vi "Best_EXP_routine_PN.vi"(0 "Psi":dbl[](array[numeric])=[39.123683, 43.320663, 43.862043], 1 "U":dbl[](array[numeric])=[2.0, 8.0, 14.0]) -> (2 "k1":dbl=0.34133317712959194 format="%#_18g", 3 "k2":dbl=0.6826663542590655 format="%#_18g", 4 "k3":dbl=1.001827918761284 format="%#_18g")   [LabVIEW 2011]
uses:
  <vilib>/Analysis/7linalg.llb/Solve Linear Equations (single right hand).vi
  <vilib>/Analysis/baseanly.llb/Real A x B.vi
  <vilib>/Analysis/Matrix/Numeric/Conversions/Array To Matrix - RA2.vi
  <vilib>/Analysis/7linalg.llb/Real Transpose Matrix.vi
  <vilib>/Analysis/baseanly.llb/Real Inverse Matrix.vi
  <vilib>/Analysis/baseanly.llb/A x Vector.vi
  <vilib>/Analysis/7linalg.llb/Solve Linear Eqs (General).vi
  <vilib>/Analysis/7linalg.llb/Solve Linear Eqs (Gen, single right hand).vi
  <vilib>/Analysis/NI_AALPro.lvlib
  <vilib>/Analysis/NI_AALBase.lvlib
  <vilib>/Analysis/Matrix/NI_Matrix.lvlib
panel:
  out "RMS err in Psi (deg)":dbl format="%#_3f"
  out "abs rel. err.":dbl[](array[numeric])=[8.183561742955495e-13, 9.91069659411527e-13, 7.387243401349263e-13] format="%#.6e"
  out "NLR against data":cluster{dbl[], "U":dbl[]}[](graph)=[{[0.0, 0.5, 1.0, 1.5, 2.0, 2.5, 3.0, 3.5, 4.0, 4.5, 5.0, 5.5, 6.0, 6.5, 7.0, 7.5, 8.0, 8.5, 9.0, 9.5, 10.0, 10.5, 11.0, 11.5, 12.0, 12.5, 13.0, 13.5, 14.0, 14.5, 15.0, 15.5, 16.0, 16.5, 17.0, 17.5, 18.0, 18.5, 19.0, 19.5, 20.0, 20.5, 21.0, 21.5, 22.0, 22.5, 23.0, 23.5, 24.0, 24.5, 25.0], "U"=[34.40562377077051, 35.90189055215256, 37.16339700573876, 38.22697641032175, 39.12368300000057, 39.87969868111344, 40.51709748766539, 41.05449009570734, 41.50756721510195, 41.88955772454882, 42.21161492642749, 42.483142199270226, 42.7120675562172, 42.90507512597115, 43.067800314998415, 43.204994349293095, 43.32066299997076, 43.418183543180774, 43.50040336931568, 43.56972312069458, 43.62816678516243, 43.677440792187646, 43.71898383693729, 43.754008887085696, 43.78353859886516, 43.8084351764313, 43.829425546372484, 43.847122582404715, 43.86204299996782, 43.87462244320632, 43.885228204842775, 43.89416995033634, 43.901708759449, 43.90806474921387, 43.91342350087974, 43.91794147848491, 43.921750597271085, 43.92496207532501, 43.92766968090778, 43.92995247028661, 43.93187709600804, 43.93349975300914, 43.934867819388955, 43.93602123974724, 43.936993691480964, 43.93781356809198, 43.93850480821628, 43.939087594580734, 43.9395789432954, 43.93999320068734, 43.940342462182606]}, {[2.0, 8.0, 14.0], "U"=[39.123683, 43.320663, 43.862043]}]
  in  "k3_0":dbl=1.0
  in  "k2_0":dbl=0.1
  in  "k1_0":dbl=0.1
  in  "show iters\ngraphically":bool
  in  "tol.":dbl=1e-12
  in  "max. iter":i32=1000
  in  "retardation":dbl=0.5
  out "Iterations":i32=37
  # "Linearise by Taylor series up to first order."
  # "r is the retardation 0...1"
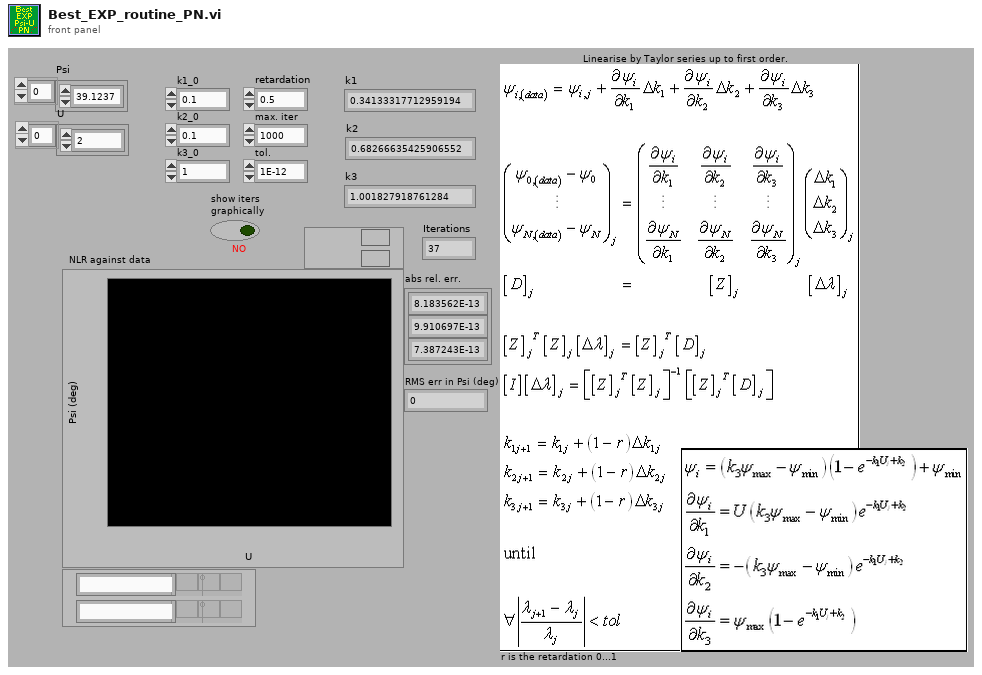
[diagram p1: front panel]
types:
  T1 = typedef "NI_Matrix.lvlib/RealMatrix.ctl" = dbl[][]
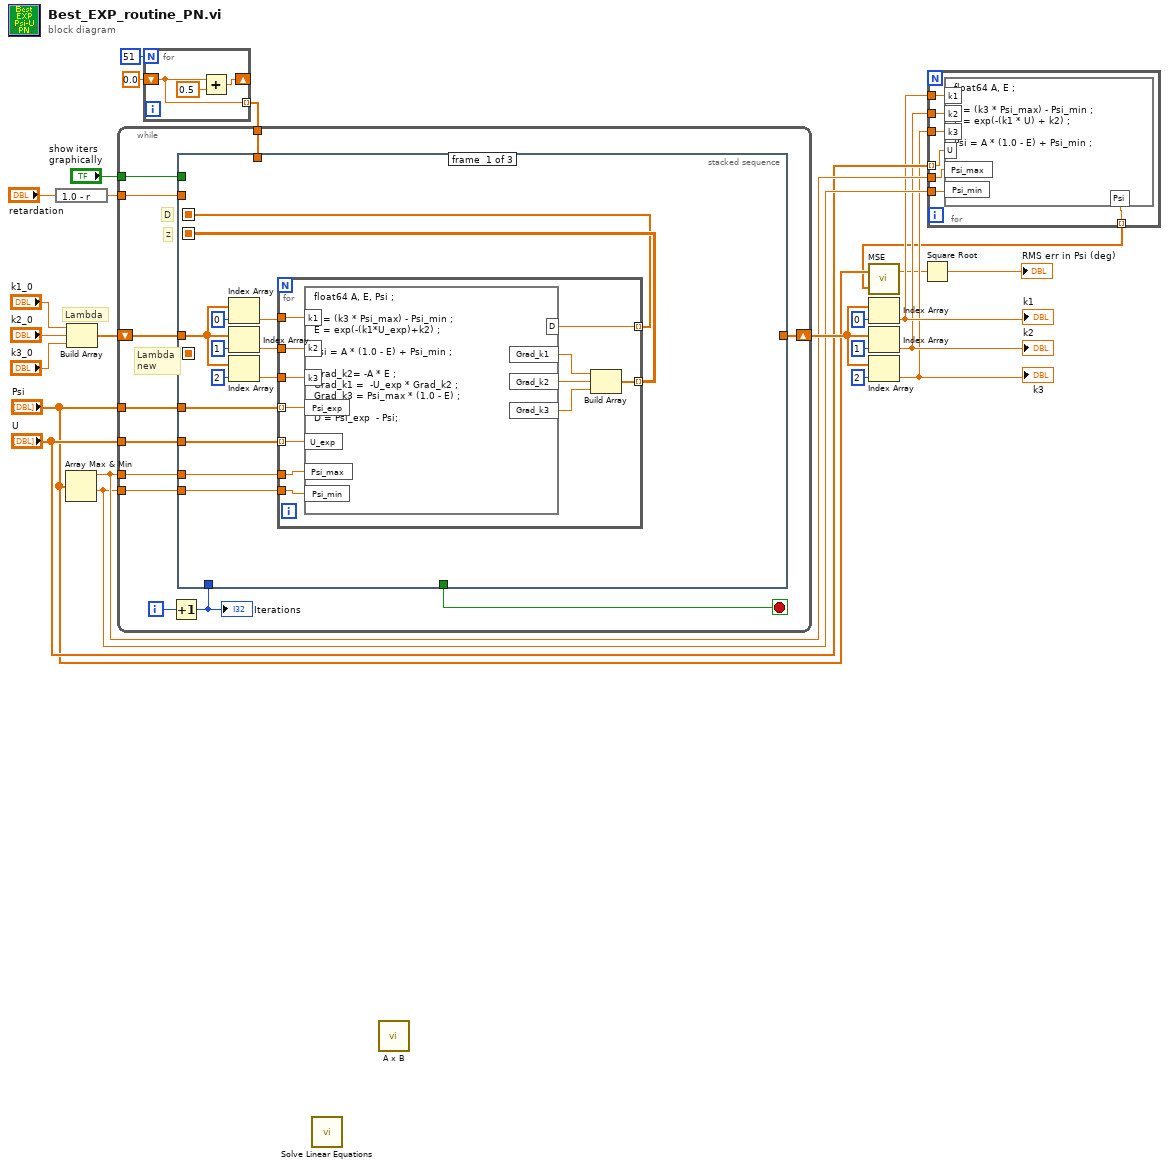
[diagram p0: block diagram]
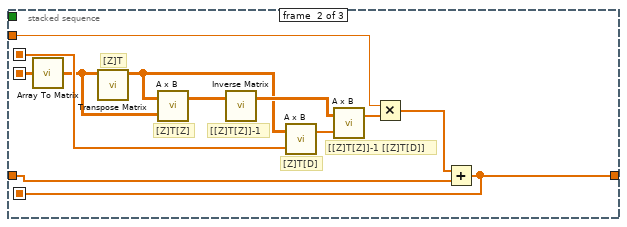
[diagram p2: hidden frame]
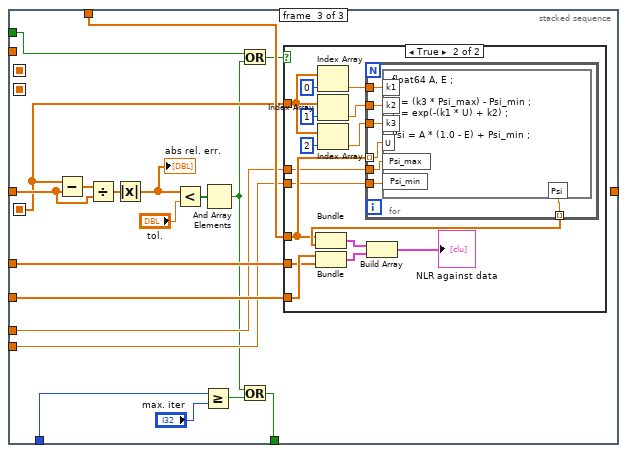
[diagram p3: hidden frame]
diagram:
  # "Lambda"
  n1 = expression code="1.0 - r"("retardation") -> (w23:dbl)
  n2 = Array Max & Min(array="Psi") -> (max value=w10:dbl, min value=w9:dbl)  [unwired: 2 out]
  n3 = Build Array("k1_0", "k2_0", "k3_0") -> (w17:dbl[])
  n4 = for {
    N: 51 ("dimension size") -> [_]
    shift-right: [w26] -> _
    shift-left: 0.0 ("element") -> [w25]
    tunnel: [w25] -> w21 mode=indexing
    n5 = Add(x=w25, y=0.5) -> (x+y=w26:dbl)
  }
  n6 = while {
    tunnel: "Psi" -> [w39]
    tunnel: "U" -> [w38]
    shift-right: [w37] -> w13
    shift-left: w17 -> [w36]
    tunnel: w23 -> [w34]
    tunnel: "show iters\ngraphically" -> [w33]
    tunnel: w21 -> [w32]
    tunnel: w10 -> [w29]
    tunnel: w9 -> [w28]
    i -> [w31]
    stop <- w35 stop-if-true
    # "Lambda\nnew"
    # "D"
    # "Z"
    n7 = Increment(x=w31) -> (x+1=w30:i32)
    "Iterations" <- w30
    n8 = stacked-sequence {
      seq-local: [w49 _ _] -> [_ w72 _]
      seq-local: [w50 _ _] -> [_ w68 _]
      seq-local: [_ w65 _] -> [_ _ w82]
      tunnel: w39 -> [w52 _ w91]
      tunnel: w38 -> [w51 _ w90]
      tunnel: [_ w65 _] -> w37
      tunnel: w36 -> [w42 w66 w95]
      tunnel: [_ _ w92] -> w35
      tunnel: w30 -> [_ _ w85]
      tunnel: w34 -> [_ w70 _]
      tunnel: w33 -> [_ _ w78]
      tunnel: w32 -> [_ _ w89]
      tunnel: w29 -> [w41 _ w81]
      tunnel: w28 -> [w40 _ w80]
      frame #0 {
        n9 = Index Array(array=w42, index=0) -> (element=w45:dbl)
        n10 = Index Array(array=w42, index=1) -> (element=w44:dbl)
        n11 = Index Array(array=w42, index=2) -> (element=w43:dbl)
        n12 = for {
          tunnel: w52 -> [w64] mode=indexing
          tunnel: w51 -> [w63] mode=indexing
          tunnel: [w59] -> w50 mode=indexing
          tunnel: [w58] -> w49 mode=indexing
          tunnel: w45 -> [w57]
          tunnel: w44 -> [w56]
          tunnel: w43 -> [w55]
          tunnel: w41 -> [w54]
          tunnel: w40 -> [w53]
          n13 = formula code="float64 A, E, Psi ;\n\nA = (k3 * Psi_max) - Psi_min ;\nE = exp(-(k1*U_exp)+k2) ;\n\nPsi = A * (1.0 - E) + Psi_min ;\n\nGrad_k2= -A * E ;\nGrad_k1 =  -U_exp * Grad_k2 ;\nGrad_k3 = Psi_max * (1.0 - E) ;\n\nD = Psi_exp  - Psi;"("Psi_exp"=w64, "U_exp"=w63, "k1"=w57, "k2"=w56, "k3"=w55, "Psi_max"=w54, "Psi_min"=w53) -> ("D"=w58:dbl, "Grad_k1"=w62:dbl, "Grad_k2"=w61:dbl, "Grad_k3"=w60:dbl)
          n14 = Build Array(w62, w61, w60) -> (w59:dbl[])
        }
      }
      frame #1 {
        # "[[Z]T[Z]]-1 [[Z]T[D]]"
        # "[Z]T[D]"
        # "[[Z]T[Z]]-1"
        # "[Z]T[Z]"
        # "[Z]T"
        n15 = call-poly <vilib>:"Array To Matrix.vi"("Real 2D Array"=w68) -> ("Real Matrix"=w69:T1)
        n16 = call-poly <vilib>:"Transpose Matrix.vi"("Input Matrix"=w69) -> ("Matrix Transpose"=w73:T1)  [unwired: 10 out]
        n17 = call-poly <vilib>:"A x B.vi"("B"=w69, "A"=w73) -> ("A x B"=w76:T1)  [unwired: 1 out]
        n18 = call-poly <vilib>:"Inverse Matrix.vi"("Input Matrix"=w76) -> ("Inverse Matrix"=w75:T1)  [unwired: 1 in, 1 out]
        n19 = call-poly <vilib>:"A x B.vi"("Vector"=w72, "A"=w73) -> ("A x Vector"=w74:dbl[])  [unwired: 1 out]
        n20 = call-poly <vilib>:"A x B.vi"("Vector"=w74, "A"=w75) -> ("A x Vector"=w71:dbl[])  [unwired: 1 out]
        n21 = Multiply(x=w70, y=w71) -> (x*y=w67:dbl[])
        n22 = Add(x=w67, y=w66) -> (x+y=w65:dbl[])
      }
      frame #2 {
        n23 = Subtract(x=w82, y=w95) -> (x-y=w86:dbl[])
        n24 = Divide(x=w86, y=w95) -> (x/y=w84:dbl[])
        n25 = Absolute Value(x=w84) -> (abs(x)=w83:dbl[])
        "abs rel. err." <- w83
        n26 = Less?(x=w83, y="tol.") -> (x < y?=w87:bool[])
        n27 = Greater Or Equal?(x=w85, y="max. iter") -> (x >= y?=w93:bool)
        n28 = And Array Elements(Boolean array=w87) -> (logical AND=w77:bool)
        n29 = Or(x=w78, y=w77) -> (x .or. y?=w79:bool)
        n30 = Or(x=w77, y=w93) -> (x .or. y?=w92:bool)
        n31 = case shown="True" w79 {
          tunnel: w91 -> [_ w108]
          tunnel: w90 -> [_ w109]
          tunnel: w89 -> [_ w99]
          tunnel: w82 -> [_ w104]
          tunnel: w81 -> [_ w98]
          tunnel: w80 -> [_ w97]
          frame False {
          }
          frame True {
            n32 = Bundle("U"=w109, "Psi"=w108) -> (w111:cluster{"U":dbl[], "Psi":dbl[]})  [unwired: 1 out]
            n33 = Index Array(array=w104, index=0) -> (element=w102:dbl)
            n34 = Index Array(array=w104, index=1) -> (element=w101:dbl)
            n35 = Index Array(array=w104, index=2) -> (element=w100:dbl)
            n36 = for {
              tunnel: [w118] -> w103 mode=indexing
              tunnel: w102 -> [w117]
              tunnel: w101 -> [w116]
              tunnel: w100 -> [w115]
              tunnel: w99 -> [w114] mode=indexing
              tunnel: w98 -> [w113]
              tunnel: w97 -> [w112]
              n37 = formula code="float64 A, E ;\n\nA = (k3 * Psi_max) - Psi_min ;\nE = exp(-(k1 * U) + k2) ;\n\nPsi = A * (1.0 - E) + Psi_min ;"("U"=w114, "k1"=w117, "k2"=w116, "k3"=w115, "Psi_max"=w113, "Psi_min"=w112) -> ("Psi"=w118:dbl)
            }
            n38 = Bundle(w99, w103) -> (w110:cluster{dbl[], dbl[]})  [unwired: 1 out]
            n39 = Build Array(w110, w111) -> (→"NLR against data":cluster{"U":dbl[], "Psi":dbl[]}[])
          }
        }
      }
    }
  }
  n40 = call-poly <vilib>:"Solve Linear Equations.vi"() -> ()  [unwired: 3 in, 2 out]
  n41 = call-poly <vilib>:"A x B.vi"() -> ()  [unwired: 2 in, 2 out]
  n42 = Index Array(array=w13, index=0) -> (element=w7:dbl)
  "k1" <- w7
  n43 = Index Array(array=w13, index=1) -> (element=w6:dbl)
  "k2" <- w6
  n44 = Index Array(array=w13, index=2) -> (element=w5:dbl)
  "k3" <- w5
  n45 = for {
    tunnel: [w125] -> w1 mode=indexing
    tunnel: w6 -> [w124]
    tunnel: w5 -> [w123]
    tunnel: "U" -> [w122] mode=indexing
    tunnel: w10 -> [w121]
    tunnel: w9 -> [w120]
    tunnel: w7 -> [w119]
    n46 = formula code="float64 A, E ;\n\nA = (k3 * Psi_max) - Psi_min ;\nE = exp(-(k1 * U) + k2) ;\n\nPsi = A * (1.0 - E) + Psi_min ;"("U"=w122, "k1"=w119, "k2"=w124, "k3"=w123, "Psi_max"=w121, "Psi_min"=w120) -> ("Psi"=w125:dbl)
  }
  n47 = call <vilib>:"MSE.vi"("X Values"=w1, "Y Values"="Psi") -> ("mse"=w4:dbl)  [unwired: 1 out]
  n48 = Square Root(x=w4) -> (sqrt(x)=→"RMS err in Psi (deg)":dbl)
